vi "getDomainReadType.vi"(8 "error in (no error)":errorcluster, 11 "IMultiReaderBuilder in":refnum<class "IMultiReaderBuilder.lvclass">) -> (0 "error out":errorcluster, 2 "SampleType out":T1 items=["daqSampleTypeInvalid", "daqSampleTypeFloat32", "daqSampleTypeFloat64", "daqSampleTypeUInt8", "daqSampleTypeInt8", "daqSampleTypeUInt16", "daqSampleTypeInt16", "daqSampleTypeUInt32", "daqSampleTypeInt32", "daqSampleTypeUInt64", "daqSampleTypeInt64", "daqSampleTypeRangeInt64", "daqSampleTypeComplexFloat32", "daqSampleTypeComplexFloat64", "daqSampleTypeBinary", "daqSampleTypeString", "daqSampleTypeStruct", "daqSampleTypeNull", "daqSampleType_count"], 3 "IMultiReaderBuilder out":refnum<class "IMultiReaderBuilder.lvclass">)   [LabVIEW 2022 SP3, in "openDAQ.lvlib" / "IBaseObject.lvlib" / "IMultiReaderBuilder.lvlib" / "IMultiReaderBuilder.lvclass"]
uses:
  <instrlib>/openDAQ/Public/Classes/IMultiReaderBuilder/IMultiReaderBuilder.lvclass
  <instrlib>/openDAQ/Public/Classes/IMultiReaderBuilder/IMultiReaderBuilder.lvclass/IMultiReaderBuilder.ctl
  <instrlib>/openDAQ/Binaries/Windows/x86/copendaq32.dll
  <instrlib>/openDAQ/Public/TypeDef/daqSampleType.ctl
  <instrlib>/openDAQ/openDAQ.lvlib
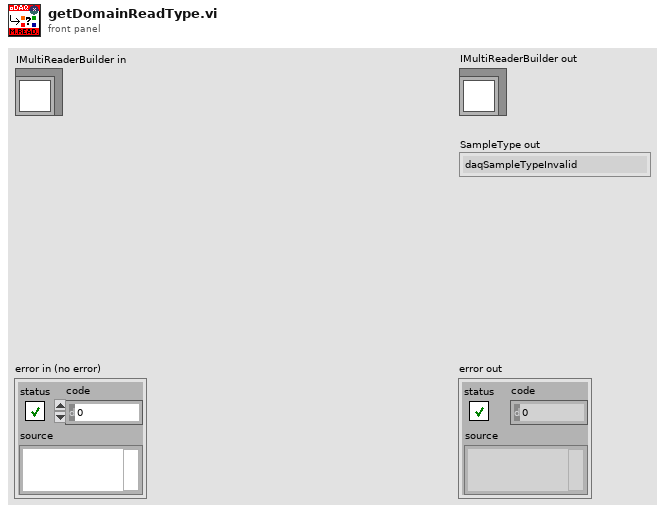
[diagram p1: front panel]
types:
  T1 = typedef "openDAQ.lvlib/daqSampleType.ctl" = u16
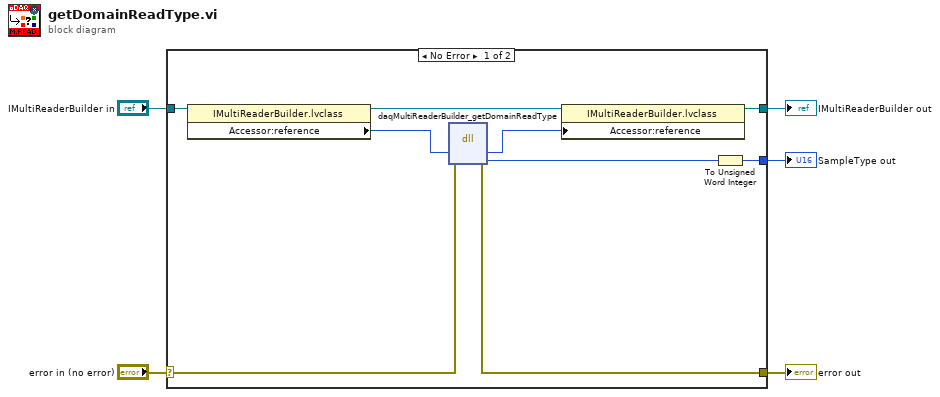
[diagram p0: block diagram]
diagram:
  n1 = case shown="No Error" "error in (no error)" {
    selector: "error in (no error)" -> [w13 w16]
    tunnel: [w12 w16] -> w4
    tunnel: [w10 w15] -> w2
    tunnel: "IMultiReaderBuilder in" -> [w14 w15]
    tunnel: [w6 _] -> w1
    frame No Error {
      n2 = property class="IMultiReaderBuilder.lvclass"(reference=w14) -> (reference out=w11:refnum<class "IMultiReaderBuilder.lvclass">, "Accessor:reference"=w9:i64)  [unwired: 1 in, 1 out]
      n3 = dll-call lib="C:/Program Files (x86)/National Instruments/LabVIEW 2022/instr.lib/openDAQ/Binaries/Windows/x86/copendaq*.*" fn="daqMultiReaderBuilder_getDomainReadType"(error in=w13, "builder"=w9) -> (error out=w12:errorcluster, "builder"=w8:i64, "readType"=w7:i64)  [unwired: 4 in, 1 out]
      n4 = property class="IMultiReaderBuilder.lvclass"(reference=w11, "Accessor:reference"=w8) -> (reference out=w10:refnum<class "IMultiReaderBuilder.lvclass">)  [unwired: 1 in, 1 out]
      n5 = To Unsigned Word Integer(number=w7) -> (unsigned 16bit integer=w6:u16)
    }
    frame Error {
    }
  }
  "error out" <- w4
  "IMultiReaderBuilder out" <- w2
  "SampleType out" <- w1
